vi "Actor Core2.vi"(8 "error in":errorcluster, 11 "InterferometryUI in":refnum<class "InterferometryUI.lvclass">) -> (0 "error out":errorcluster, 3 "Actor out":refnum<class "Actor.lvclass">)   [LabVIEW 2023, in "InterferometryUI.lvlib" / "InterferometryUI.lvclass"]
doc: "(<B>Filename</B>: Actor Framework.lvlib:Actor.lvclass:Actor Core.vi)\n\nReceives messages to the actor, reacts to them, and initiates any error handling that may shut the actor down.\n\nDescendant classes may override this VI to append parallel tasks for the actor to complete while it handles messages. Overrides use the Call Parent Class Method node."
uses:
  InterferometryUI.lvclass
  InterferometryUI.lvclass/InterferometryUI.ctl
  <vilib>/ActorFramework/Actor/Actor.lvclass
  <vilib>/ActorFramework/Stop Msg/Stop Msg.lvclass
  ArduinoTranslationStageUI/ArduinoTranslationStageActor/ArduinoTranslationStage Actor/ArduinoTranslationStage.lvclass
  ConcreteClasses/ConcreteInstrumentClasses/CameraClasses/ZWO_ASI_LV/ZWO_ASI/ZWO_ASI.lvclass
  ArduinoTranslationStageUI/ArduinoTranslationStageActor/ArduinoTranslationStage Messages/MoveBySteps Msg/MoveBySteps Msg.lvclass
  ConcreteClasses/ConcreteInstrumentClasses/CameraClasses/ZWO_ASI_LV/ZWO_ASI Messages/StartCapture Msg/StartCapture Msg.lvclass
  ConcreteClasses/ConcreteInstrumentClasses/CameraClasses/ZWO_ASI_LV/ZWO_ASI Messages/StopCapture Msg/StopCapture Msg.lvclass
  ConcreteClasses/ConcreteInstrumentClasses/CameraClasses/ZWO_ASI_LV/ZWO_ASI Messages/OpenCamera Msg/OpenCamera Msg.lvclass
  ArduinoTranslationStageUI/ArduinoTranslationStageActor/ArduinoTranslationStage Messages/Init Msg/Init Msg.lvclass
  Applications/National Instruments/LabVIEW 2023 64-bit/vi.lib/ActorFramework/Actor/Actor.lvclass
  Users/alexandrosspiliotis/Documents/LV_DAQ_Project/UIs/ArduinoTranslationStageUI/ArduinoTranslationStageActor/ArduinoTranslationStage Actor/ArduinoTranslationStage.lvclass
  Users/alexandrosspiliotis/Documents/LV_DAQ_Project/Interfaces/InitDeinitInterface/InitDeinit/InitDeinit.lvclass
  Users/alexandrosspiliotis/Documents/LV_DAQ_Project/Interfaces/AbstractInstrumentClasses/StepperMotorControllers_LV/StepperMotorController/StepperMotorController.lvclass
  Users/alexandrosspiliotis/Documents/LV_DAQ_Project/Interfaces/AbstractInstrumentClasses/TranslationStages_LV/TranslationStageInterface/TranslationStagesInterface.lvclass
  Users/alexandrosspiliotis/Documents/LV_DAQ_Project/ConcreteClasses/ConcreteInstrumentClasses/CameraClasses/ZWO_ASI_LV/ZWO_ASI/ZWO_ASI.lvclass
  Users/alexandrosspiliotis/Documents/LV_DAQ_Project/Interfaces/AbstractInstrumentClasses/Cameras_LV/CameraInterface/CameraInterface.lvclass
panel:
  in  "FileName":string
  in  "Path":path
  out "VI":refnum<vi>
  out "Image":u16[][](graph)
  in  "Exposure":dbl
  in  "Snap":bool
  in  "Live":bool
  in  "Connect Cam":bool
  in  "Connect Stepper":bool
  in  "VISA resource name":refnum<visa-resource-name>
  in  "Stop Button":bool
  in  "Direction":enum16{"Forward", "Backwards"}(ring)
  in  "Polarity":enum16{"Positive", "Negative"}(ring)
  in  "Move Stepper":bool
  in  "Step Time (us)":u32(slide)=100 min=100 step=10 scale=100.0..10000.0
  in  "Steps":u32(slide)=1 min=1 max=10000 step=1 scale=1.0..10000.0
  in  "Scan Segments":u32(slide) max=100 step=1 scale=0.0..100.0
  in  "Scan":bool
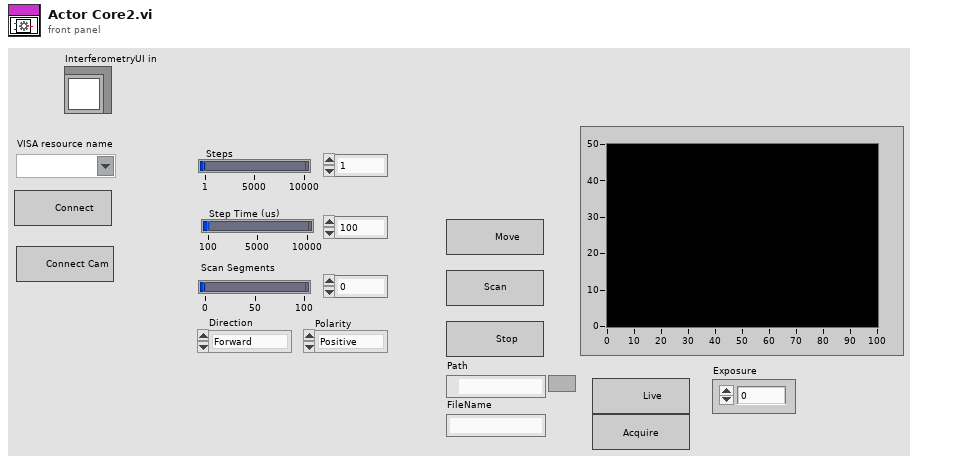
[diagram p1: front panel]
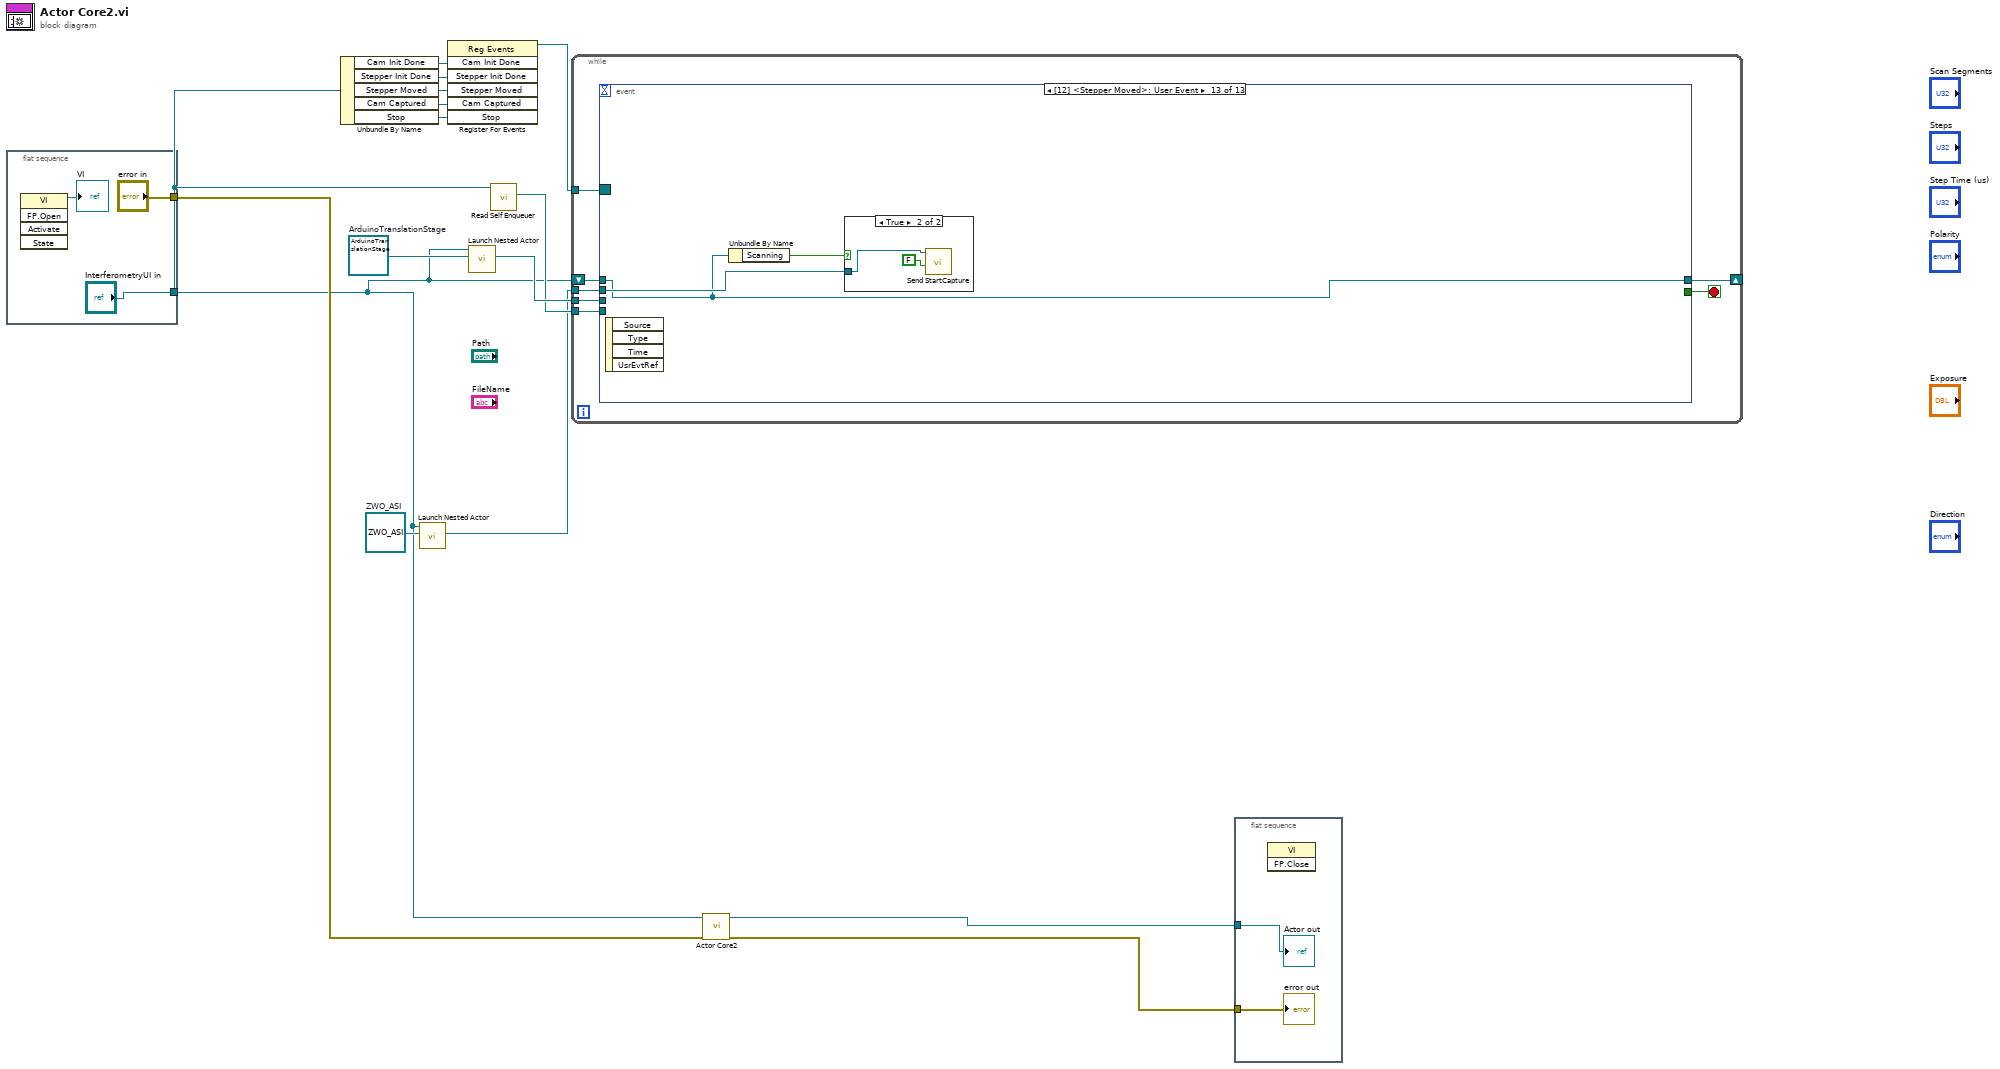
[diagram p0: block diagram]
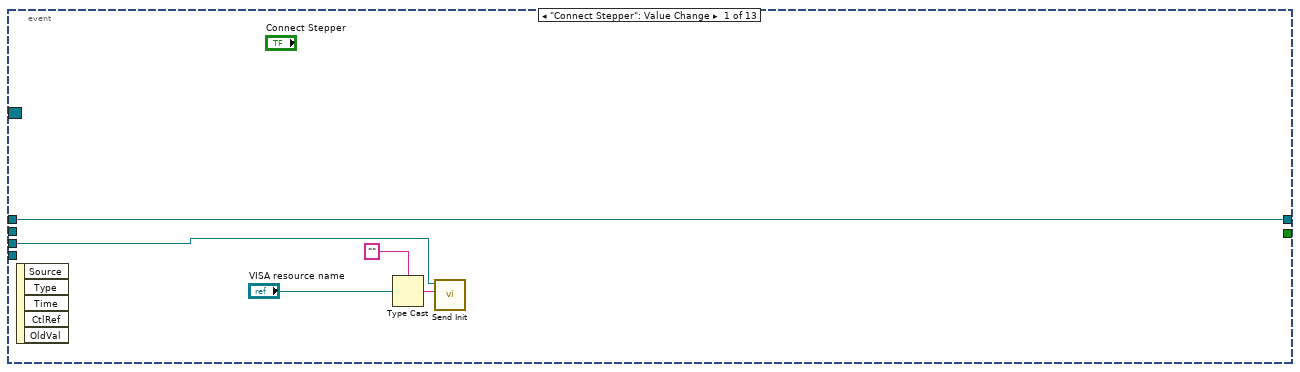
[diagram p2: hidden frame]
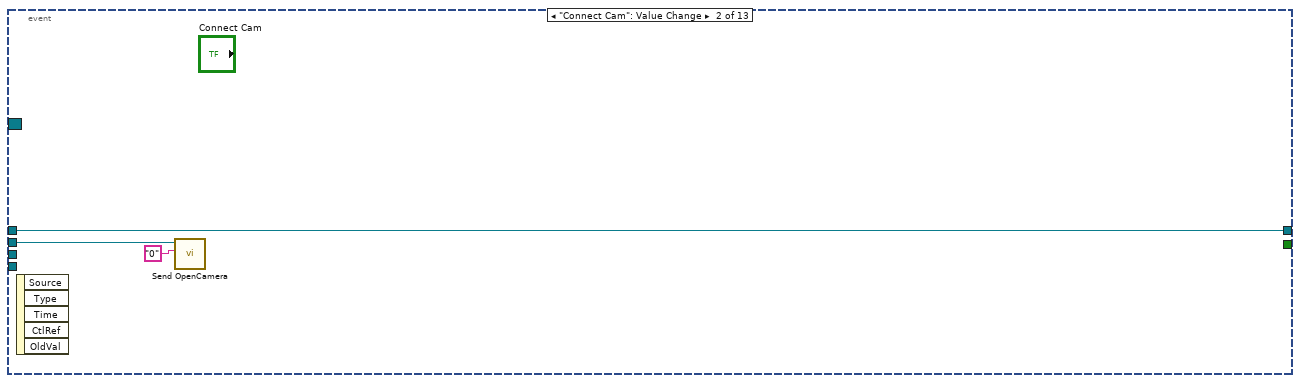
[diagram p3: hidden frame]
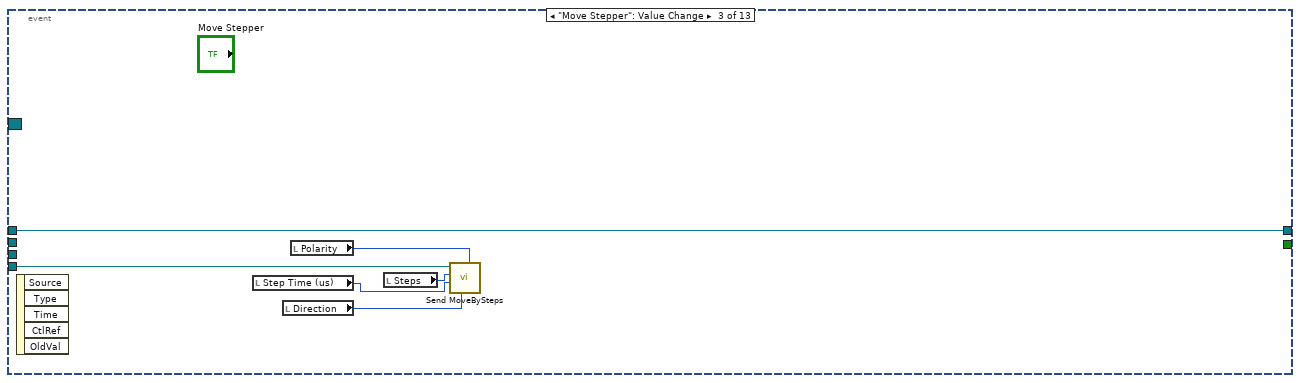
[diagram p4: hidden frame]
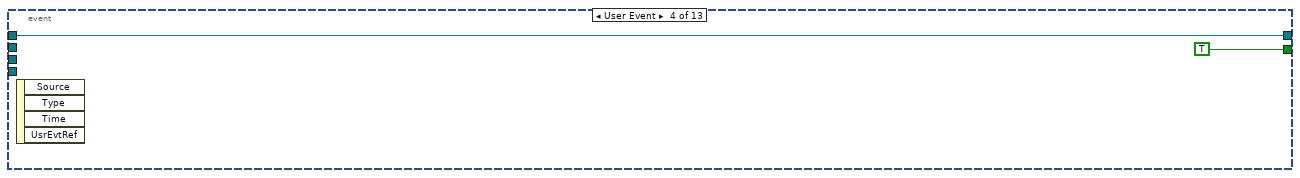
[diagram p5: hidden frame]
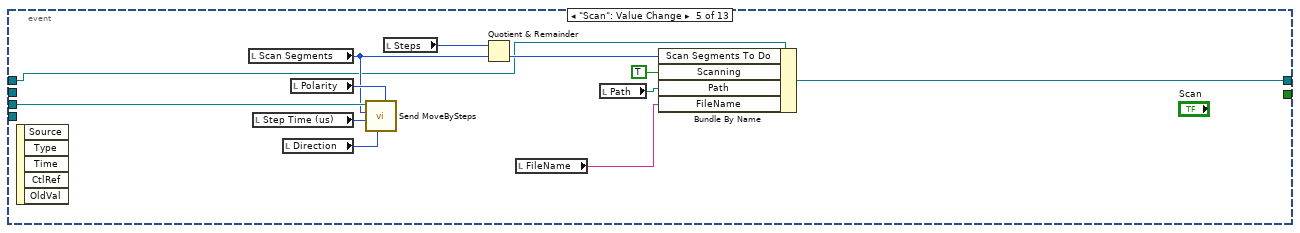
[diagram p6: hidden frame]
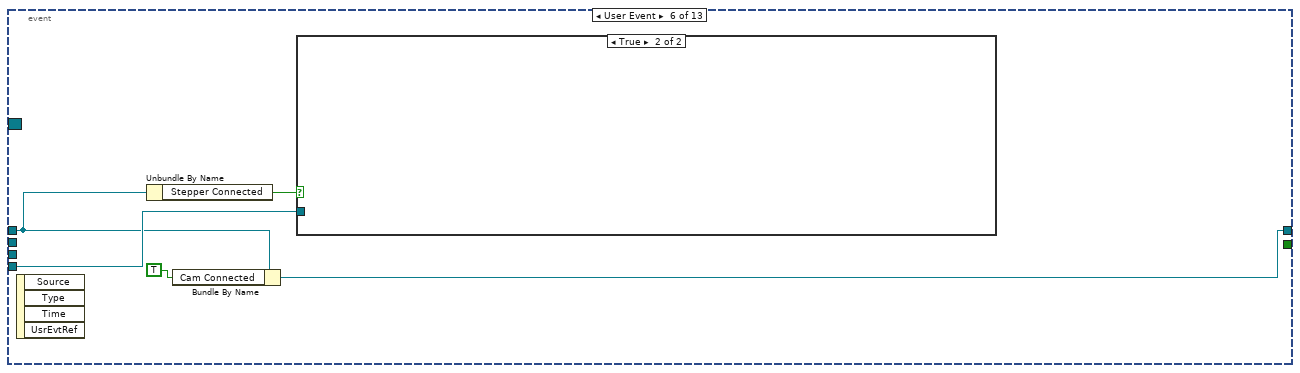
[diagram p7: hidden frame]
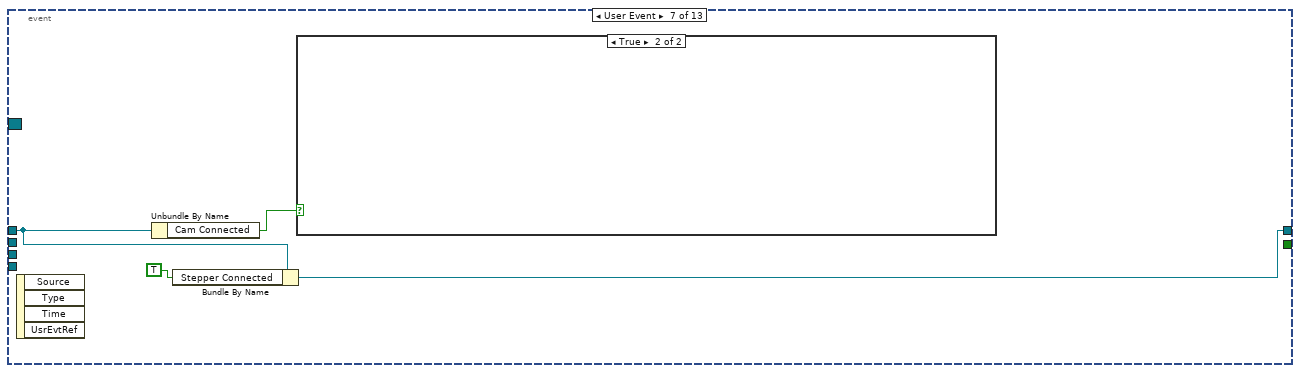
[diagram p9: hidden frame]
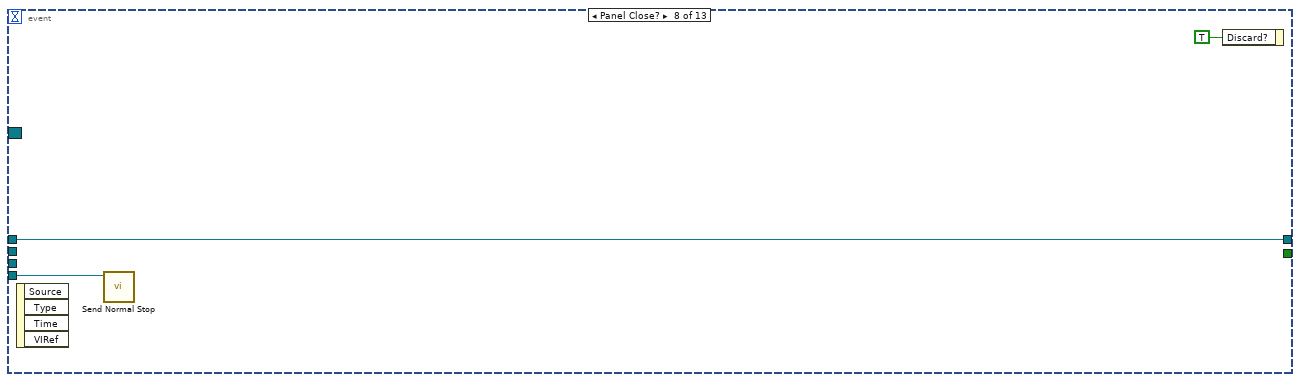
[diagram p11: hidden frame]
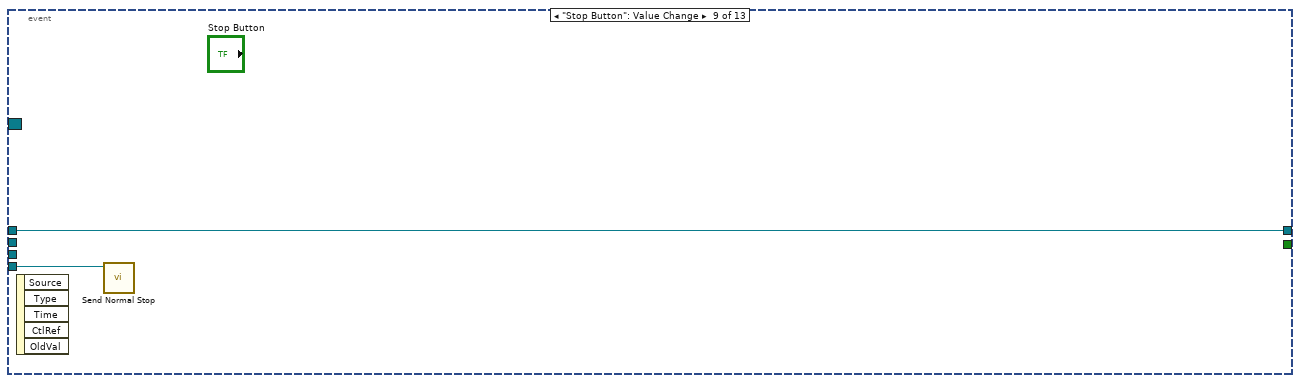
[diagram p12: hidden frame]
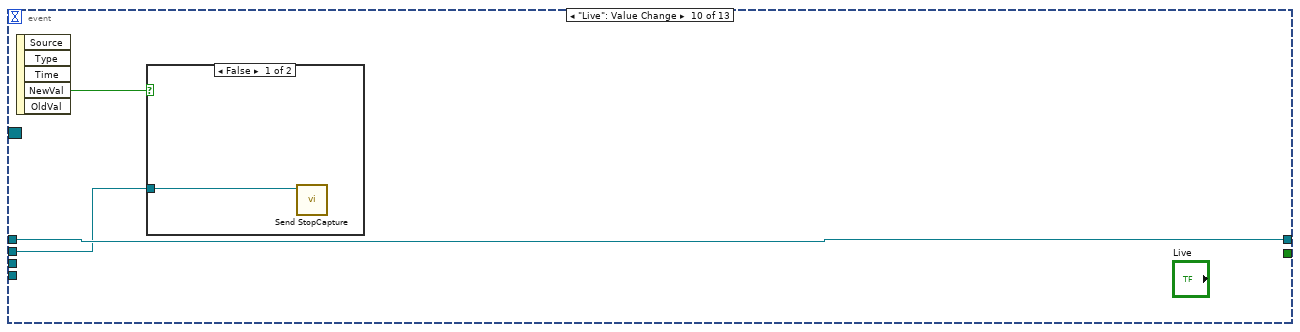
[diagram p13: hidden frame]
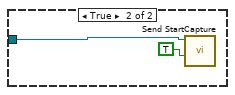
[diagram p14: hidden frame]
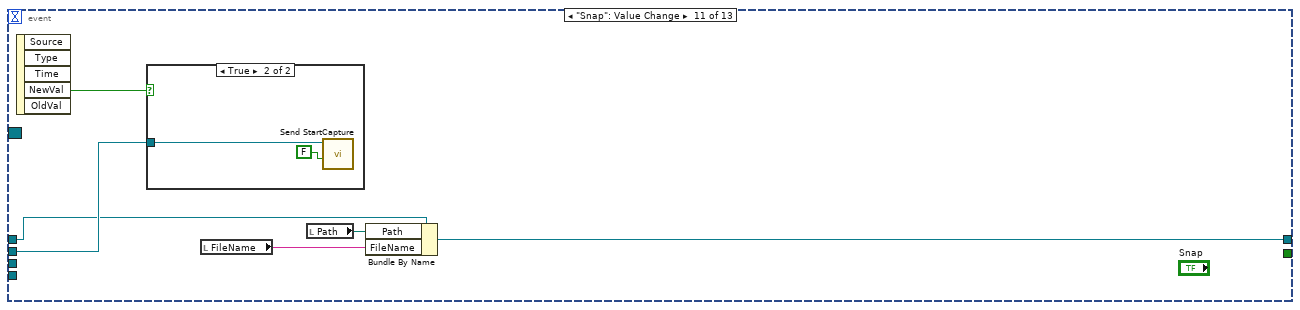
[diagram p15: hidden frame]
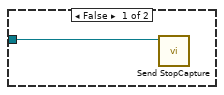
[diagram p16: hidden frame]
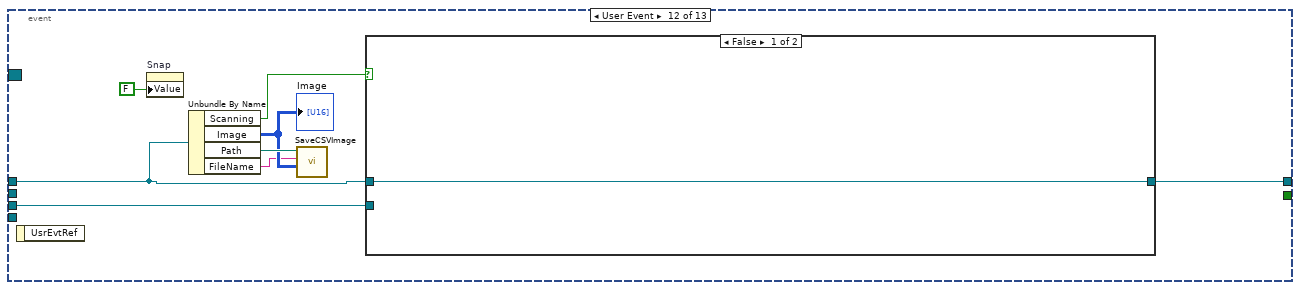
[diagram p17: hidden frame]
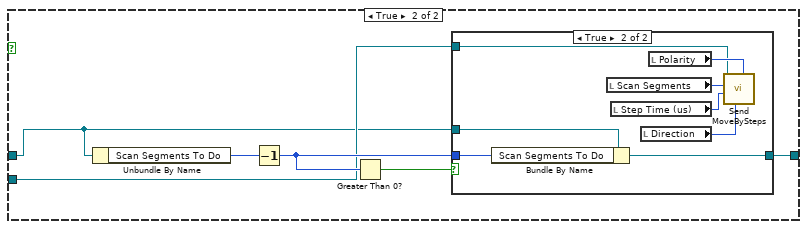
[diagram p18: hidden frame]
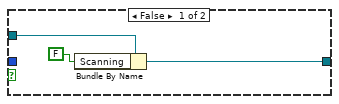
[diagram p19: hidden frame]
diagram:
  w8 = refnum<class "ZWO_ASI.lvclass"> refnum  # ZWO_ASI
  w9 = refnum<class "ArduinoTranslationStage.lvclass"> refnum  # ArduinoTranslationStage
  n1 = flat-sequence {
    tunnel: ["error in"] -> w13
    tunnel: ["InterferometryUI in"] -> w1
    frame #0 {
      n2 = invoke class="VI" method="FP.Open"() -> (reference out=→"VI":refnum<vi>)  [unwired: 5 in, 4 out]
    }
  }
  n3 = Unbundle By Name(w1) -> ("Cam Init Done"=w6:refnum<user-event>, "Stepper Init Done"=w5:refnum<user-event>, "Stepper Moved"=w4:refnum<user-event>, "Cam Captured"=w3:refnum<user-event>, "Stop"=w2:refnum<user-event>)
  n4 = call <vilib>:"Launch Nested Actor.vi"("Nested Actor"=w8, "Caller Actor in"=w1) -> ("Nested Actor's Enqueuer"=w10:refnum<class "Message Enqueuer.lvclass">)  [unwired: 7 in, 2 out]
  n5 = register-events(w6, w5, w4, w3, w2) -> (reference out=w7:refnum<event-registration>)  [unwired: 2 in, 1 out]
  n6 = call <vilib>:"Launch Nested Actor.vi"("Nested Actor"=w9, "Caller Actor in"=w1) -> ("Nested Actor's Enqueuer"=w12:refnum<class "Message Enqueuer.lvclass">)  [unwired: 7 in, 2 out]
  n7 = call <vilib>:"Read Self Enqueuer.vi"("Actor"=w1) -> ("Self Enqueuer"=w11:refnum<class "Message Enqueuer.lvclass">)  [unwired: 10 in]
  n8 = while {
    tunnel: w12 -> [w22]
    tunnel: w11 -> [w23]
    tunnel: w10 -> [w19]
    shift-right: [w25] -> _
    shift-left: w1 -> [w24]
    tunnel: w7 -> [w21]
    stop <- w20 stop-if-true
    n9 = event shown="[12] <Stepper Moved>: User Event" {
      selector: w21 -> [_ _ _ _ _ _ _ _ _ _ _ _ _]
      dyn-events: _ -> [_ _ _ _ _ _ _ _ _ _ _ _ _]
      timeout: _ -> [_ _ _ _ _ _ _ _ _ _ _ _ _]
      tunnel: [w30 w33 w39 w41 w43 w56 w59 w65 w67 w70 w74 w83 w109] -> w25
      tunnel: w24 -> [w30 w33 w39 w41 w42 w54 w60 w65 w67 w70 w75 w88 w109]
      tunnel: w23 -> [_ _ w34 _ _ w57 _ w64 w66 _ _ _ _]
      tunnel: w22 -> [w27 _ _ _ w49 _ _ _ _ _ _ w89 _]
      tunnel: [_ _ _ TRUE _ _ _ _ _ _ _ _ _] -> w20
      tunnel: w19 -> [_ w32 _ _ _ _ _ _ _ w69 w79 _ w111]
      event "Connect Stepper": Value Change {
        n10 = event-data() -> ()  [unwired: 1 in, 5 out]
        n11 = Type Cast(type="", x="VISA resource name") -> (*(type *) &x=w26:string)
        n12 = call "Send Init.vi"("Address"=w26, "Message Enqueuer"=w27) -> ()  [unwired: 8 in, 2 out]
      }
      event "Connect Cam": Value Change {
        n13 = event-data() -> ()  [unwired: 1 in, 5 out]
        n14 = call "Send OpenCamera.vi"("Camera ID"="0", "Message Enqueuer"=w32) -> ()  [unwired: 8 in, 2 out]
      }
      event "Move Stepper": Value Change {
        n15 = event-data() -> ()  [unwired: 1 in, 5 out]
        n16 = local read "Step Time (us)"() -> (w37:u32)
        n17 = local read "Direction"() -> (w35:enum16{"Forward", "Backwards"})
        n18 = local read "Polarity"() -> (w36:enum16{"Positive", "Negative"})
        n19 = local read "Steps"() -> (w38:u32)
        n20 = call "Send MoveBySteps.vi"("Polarity"=w36, "Direction"=w35, "Speed"=w37, "Steps"=w38, "Message Enqueuer"=w34) -> ()  [unwired: 5 in, 2 out]
      }
      event User Event {
        n21 = event-data() -> ()  [unwired: 1 in, 4 out]
      }
      event "Scan": Value Change {
        n22 = event-data() -> ()  [unwired: 1 in, 5 out]
        n23 = local read "Scan Segments"() -> (w47:u32)
        n24 = local read "Step Time (us)"() -> (w52:u32)
        n25 = local read "Direction"() -> (w50:enum16{"Forward", "Backwards"})
        n26 = local read "Polarity"() -> (w51:enum16{"Positive", "Negative"})
        n27 = call "Send MoveBySteps.vi"("Polarity"=w51, "Direction"=w50, "Speed"=w52, "Steps"=w47, "Message Enqueuer"=w49) -> ()  [unwired: 5 in, 2 out]
        n28 = local read "Steps"() -> (w48:u32)
        n29 = Quotient & Remainder(x=w48, y=w47) -> (floor(x/y)=w46:u32)  [unwired: 1 out]
        n30 = local read "FileName"() -> (w44:string)
        n31 = local read "Path"() -> (w45:path)
        n32 = Bundle By Name(cluster=w42, "Scan Segments To Do"=w46, "Scanning"=TRUE, "Path"=w45, "FileName"=w44) -> (w43:refnum<class "InterferometryUI.lvclass">)
      }
      event User Event {
        n33 = event-data() -> ()  [unwired: 1 in, 4 out]
        n34 = Unbundle By Name(w54) -> ("Stepper Connected"=w55:bool)
        n35 = Bundle By Name(cluster=w54, "Cam Connected"=TRUE) -> (w56:refnum<class "InterferometryUI.lvclass">)
        n36 = case shown="True" w55 {
          tunnel: w57 -> [_ _]
          frame False {
          }
          frame True {
          }
        }
      }
      event User Event {
        n37 = event-data() -> ()  [unwired: 1 in, 4 out]
        n38 = Unbundle By Name(w60) -> ("Cam Connected"=w61:bool)
        n39 = Bundle By Name(cluster=w60, "Stepper Connected"=TRUE ("Cam Connected")) -> (w59:refnum<class "InterferometryUI.lvclass">)
        n40 = case shown="True" w61 {
          frame False {
          }
          frame True {
          }
        }
      }
      event Panel Close? {
        n41 = event-data() -> ()  [unwired: 1 in, 4 out]
        n42 = call <vilib>:"Send Normal Stop.vi"("Message Enqueuer"=w64) -> ()  [unwired: 10 in, 1 out]
        n43 = event-data("Discard?"=TRUE) -> ()  [unwired: 1 in, 1 out]
      }
      event "Stop Button": Value Change {
        n44 = event-data() -> ()  [unwired: 1 in, 5 out]
        n45 = call <vilib>:"Send Normal Stop.vi"("Message Enqueuer"=w66) -> ()  [unwired: 10 in, 1 out]
      }
      event "Live": Value Change {
        n46 = event-data() -> ("NewVal"=w68:bool)  [unwired: 1 in, 4 out]
        n47 = case shown="False" w68 {
          tunnel: w69 -> [w71 w73]
          frame False {
            n48 = call "Send StopCapture.vi"("Message Enqueuer"=w71) -> ()  [unwired: 9 in, 2 out]
          }
          frame True {
            n49 = call "Send StartCapture.vi"("Continuous"=TRUE, "Message Enqueuer"=w73) -> ()  [unwired: 8 in, 2 out]
          }
        }
      }
      event "Snap": Value Change {
        n50 = event-data() -> ("NewVal"=w78:bool)  [unwired: 1 in, 4 out]
        n51 = case shown="True" w78 {
          tunnel: w79 -> [w80 w82]
          frame False {
            n52 = call "Send StopCapture.vi"("Message Enqueuer"=w80) -> ()  [unwired: 9 in, 2 out]
          }
          frame True {
            n53 = call "Send StartCapture.vi"("Continuous"=FALSE, "Message Enqueuer"=w82) -> ()  [unwired: 8 in, 2 out]
          }
        }
        n54 = local read "FileName"() -> (w76:string)
        n55 = local read "Path"() -> (w77:path)
        n56 = Bundle By Name(cluster=w75, "Path"=w77, "FileName"=w76) -> (w74:refnum<class "InterferometryUI.lvclass">)
      }
      event User Event {
        n57 = event-data() -> ()  [unwired: 1 in, 1 out]
        n58 = property on="Snap" class="Bool (strict)"("Value"=FALSE ("Snap")) -> ()  [unwired: 2 in, 2 out]
        n59 = Unbundle By Name(w88) -> ("Scanning"=w84:bool, "Image"=w86:u16[][], "Path"=w87:path, "FileName"=w85:string)
        "Image" <- w86
        n60 = call "SaveCSVImage.vi"("Image"=w86, "FileName"=w85, "Path"=w87) -> ()  [unwired: 9 in]
        n61 = case shown="False" w84 {
          tunnel: w88 -> [w91 w92]
          tunnel: [w91 w97] -> w83
          tunnel: w89 -> [_ w94]
          frame False {
          }
          frame True {
            n62 = Unbundle By Name(w92) -> ("Scan Segments To Do"=w93:u16)
            n63 = Decrement(x=w93) -> (x-1=w96:u16)
            n64 = Greater Than 0?(x=w96) -> (x > 0?=w95:bool)
            n65 = case shown="True" w95 {
              tunnel: [w99 w105] -> w97
              tunnel: w92 -> [w98 w101]
              tunnel: w96 -> [_ w103]
              tunnel: w94 -> [_ w102]
              frame False {
                n66 = Bundle By Name(cluster=w98, "Scanning"=FALSE) -> (w99:refnum<class "InterferometryUI.lvclass">)
              }
              frame True {
                n67 = Bundle By Name(cluster=w101, "Scan Segments To Do"=w103) -> (w105:refnum<class "InterferometryUI.lvclass">)
                n68 = local read "Scan Segments"() -> (w104:u32)
                n69 = local read "Step Time (us)"() -> (w108:u32)
                n70 = local read "Direction"() -> (w106:enum16{"Forward", "Backwards"})
                n71 = local read "Polarity"() -> (w107:enum16{"Positive", "Negative"})
                n72 = call "Send MoveBySteps.vi"("Polarity"=w107, "Direction"=w106, "Speed"=w108, "Steps"=w104, "Message Enqueuer"=w102) -> ()  [unwired: 5 in, 2 out]
              }
            }
          }
        }
      }
      event User Event {
        n73 = event-data() -> ()  [unwired: 1 in, 4 out]
        n74 = Unbundle By Name(w109) -> ("Scanning"=w110:bool)
        n75 = case shown="True" w110 {
          tunnel: w111 -> [_ w113]
          frame False {
          }
          frame True {
            n76 = call "Send StartCapture.vi"("Continuous"=FALSE, "Message Enqueuer"=w113) -> ()  [unwired: 8 in, 2 out]
          }
        }
      }
    }
  }
  n77 = call-parent "Actor Core2.vi"("error in"=w13, "Actor in"=w1) -> ("error out"=w15:errorcluster, "Actor out"=w14:refnum<class "Actor.lvclass">)  [unwired: 8 in]
  n78 = flat-sequence {
    tunnel: w15 -> [w115]
    tunnel: w14 -> [w114]
    frame #0 {
      n79 = invoke class="VI" method="FP.Close"() -> ()  [unwired: 3 in, 3 out]
      "error out" <- w115
      "Actor out" <- w114
    }
  }
